vi "DPT File Setup.vi"(0 "Data File Directory":path=path "D:/Data", 1 "Test_Type:":string="HeatUP", 3 "Version In:":string="DGnn", 4 "Supply Voltage:":string(combo), 5 "error in (no error)":errorcluster, 7 "File Extension:":string="tmp", 12 "Scale Com Port":refnum<visa-resource-name>="COM1", 18 "Flow Computer Info Baro,BTUF,u,Z":string[][](array[string])) -> (11 "FileInit Cluster":T1={"Dryer Type"="NR", "TR Number"="", "Lab ID"="", "Output Stream Header"=[], "Stream Data Output"=[], "2015 Array"=[], "Dryer Test Data"=[], "Off Mode Array"=[], "Calibration Array"=[], "File Initialization Array"=[], "Load Run Number"="", "Model:"="DGnn", "Serial Number:"="DGnn", "Build:"="", "Test_Title Per TR:"="HeatUP", "Ambient Temp SetPoint:"="70", "Washer Water \nTemperature ( 60 ± 5°F ):"="60", "Frequency:"="60 HZ", "Dryness Setting:"="", "Heat Setting:"="", "Ambient RH:"="50", "Drying Cycle:"="", "Exhaust:"="NR", "Comments:"="", "Technician:"="", "Engineer:"="CraigT.", "Water Hardness (PPM)"="60", "Empty Dryer Cold Weight"="HeatUP", "Date:"="DGnn", "Version:"="DGnn", "Computer:"="1A", "Load Type"="", "Nominal Load  Weight"="", "Weights Out"={"Measured IMC"=7.0, "Actual RMC"=7.0, "RMC (Desired)"=100.0, "Bone Dry Wt(lbs)"=7.0, "Tolerance(%)"=5.0}, "Test Station:"="1A", "Heat Setting:"="", "Dryness Setting:"="", "Frequency:"="60 HZ", "Water Hardness (PPM)"="60", "Washer Water \nTemperature ( 60 ± 5°F )"="60", "Flow Computer Info Baro,BTUF,u,Z"=[], "Filename"="", "Analog Voltage Data"=[]} {"Weights Out"."Tolerance(%)" format="%0#_6g"; "Weights Out"."Bone Dry Wt(lbs)" format="%03_6g"; "Weights Out"."RMC (Desired)" format="%0#_6g"; "Weights Out"."Actual RMC" format="%03_6g"; "Weights Out"."Measured IMC" format="%0#_6g"}, 13 "Weights Out":T4={"Measured IMC"=7.0, "Actual RMC"=7.0, "RMC (Desired)"=100.0, "Bone Dry Wt(lbs)"=7.0, "Tolerance(%)"=5.0} {"Tolerance(%)" format="%0#_6g"; "Bone Dry Wt(lbs)" format="%03_6g"; "RMC (Desired)" format="%0#_6g"; "Actual RMC" format="%03_6g"; "Measured IMC" format="%0#_6g"}, 14 "FileName":path, 17 "Nominal Load  Weight":string(combo), 19 "error out":errorcluster)   [LabVIEW 2016, in "File Setup.lvlib"]
uses:
  File Setup.lvlib
  DPT Global Test Variables.vi
  Type Definition/DPT Output Dryer Information.ctl
  Custom Pallet Controls/Custom Pallet String.ctl
  Custom Pallet Controls/Custom Pallet Forward.ctl
panel:
  out "Description":string="File Name Setup"
  in  "Water Hardness (PPM)":T2
  in  "Model:":T2="DGnn"
  in  "Ambient Temp SetPoint:":T2="70"
  in  "Test_Title Per TR:":T2="HeatUP"
  in  "Engineer:":T2="CraigT."
  in  "Technician:":T2
  in  "Comments:":string
  in  "Lab ID:":T2="DGnn"
  in  "TR Number:":T2="T000000"
  in  "Load Run Number:":T2="001"
  in  "Exhaust:":string(combo)="NR"
  in  "Drying Cycle:":string(combo)
  in  "OK":T3
  in  "Serial Number:":T2="DGnn"
  in  "Ambient RH:":T2="50"
  in  "Build:":string(combo)
  in  "Heat Setting:":T2
  in  "Dryness Setting:":T2
  in  "Frequency:":T2="60 HZ"
  in  "Washer Water \nTemperature ( 60 ± 5°F ):":T2="60"
  in  "Dryer Type":string(combo)
  in  "Tab Control":enum32{"Location Data", "Output Data"}(tab)
  out "Unhandled Error":errorcluster
  out "Filename":string
  in  "Load Definition File":path=path "c:/Work/Loads.ini"
  out "Version:":string="DGnn"
  out "Computer:":string="1A"
  in  "Read Scale for IMC":bool
  out "Load Type":string(combo)
  out "Date:":string="DGnn"
  in  "Test Station:":string="1A"
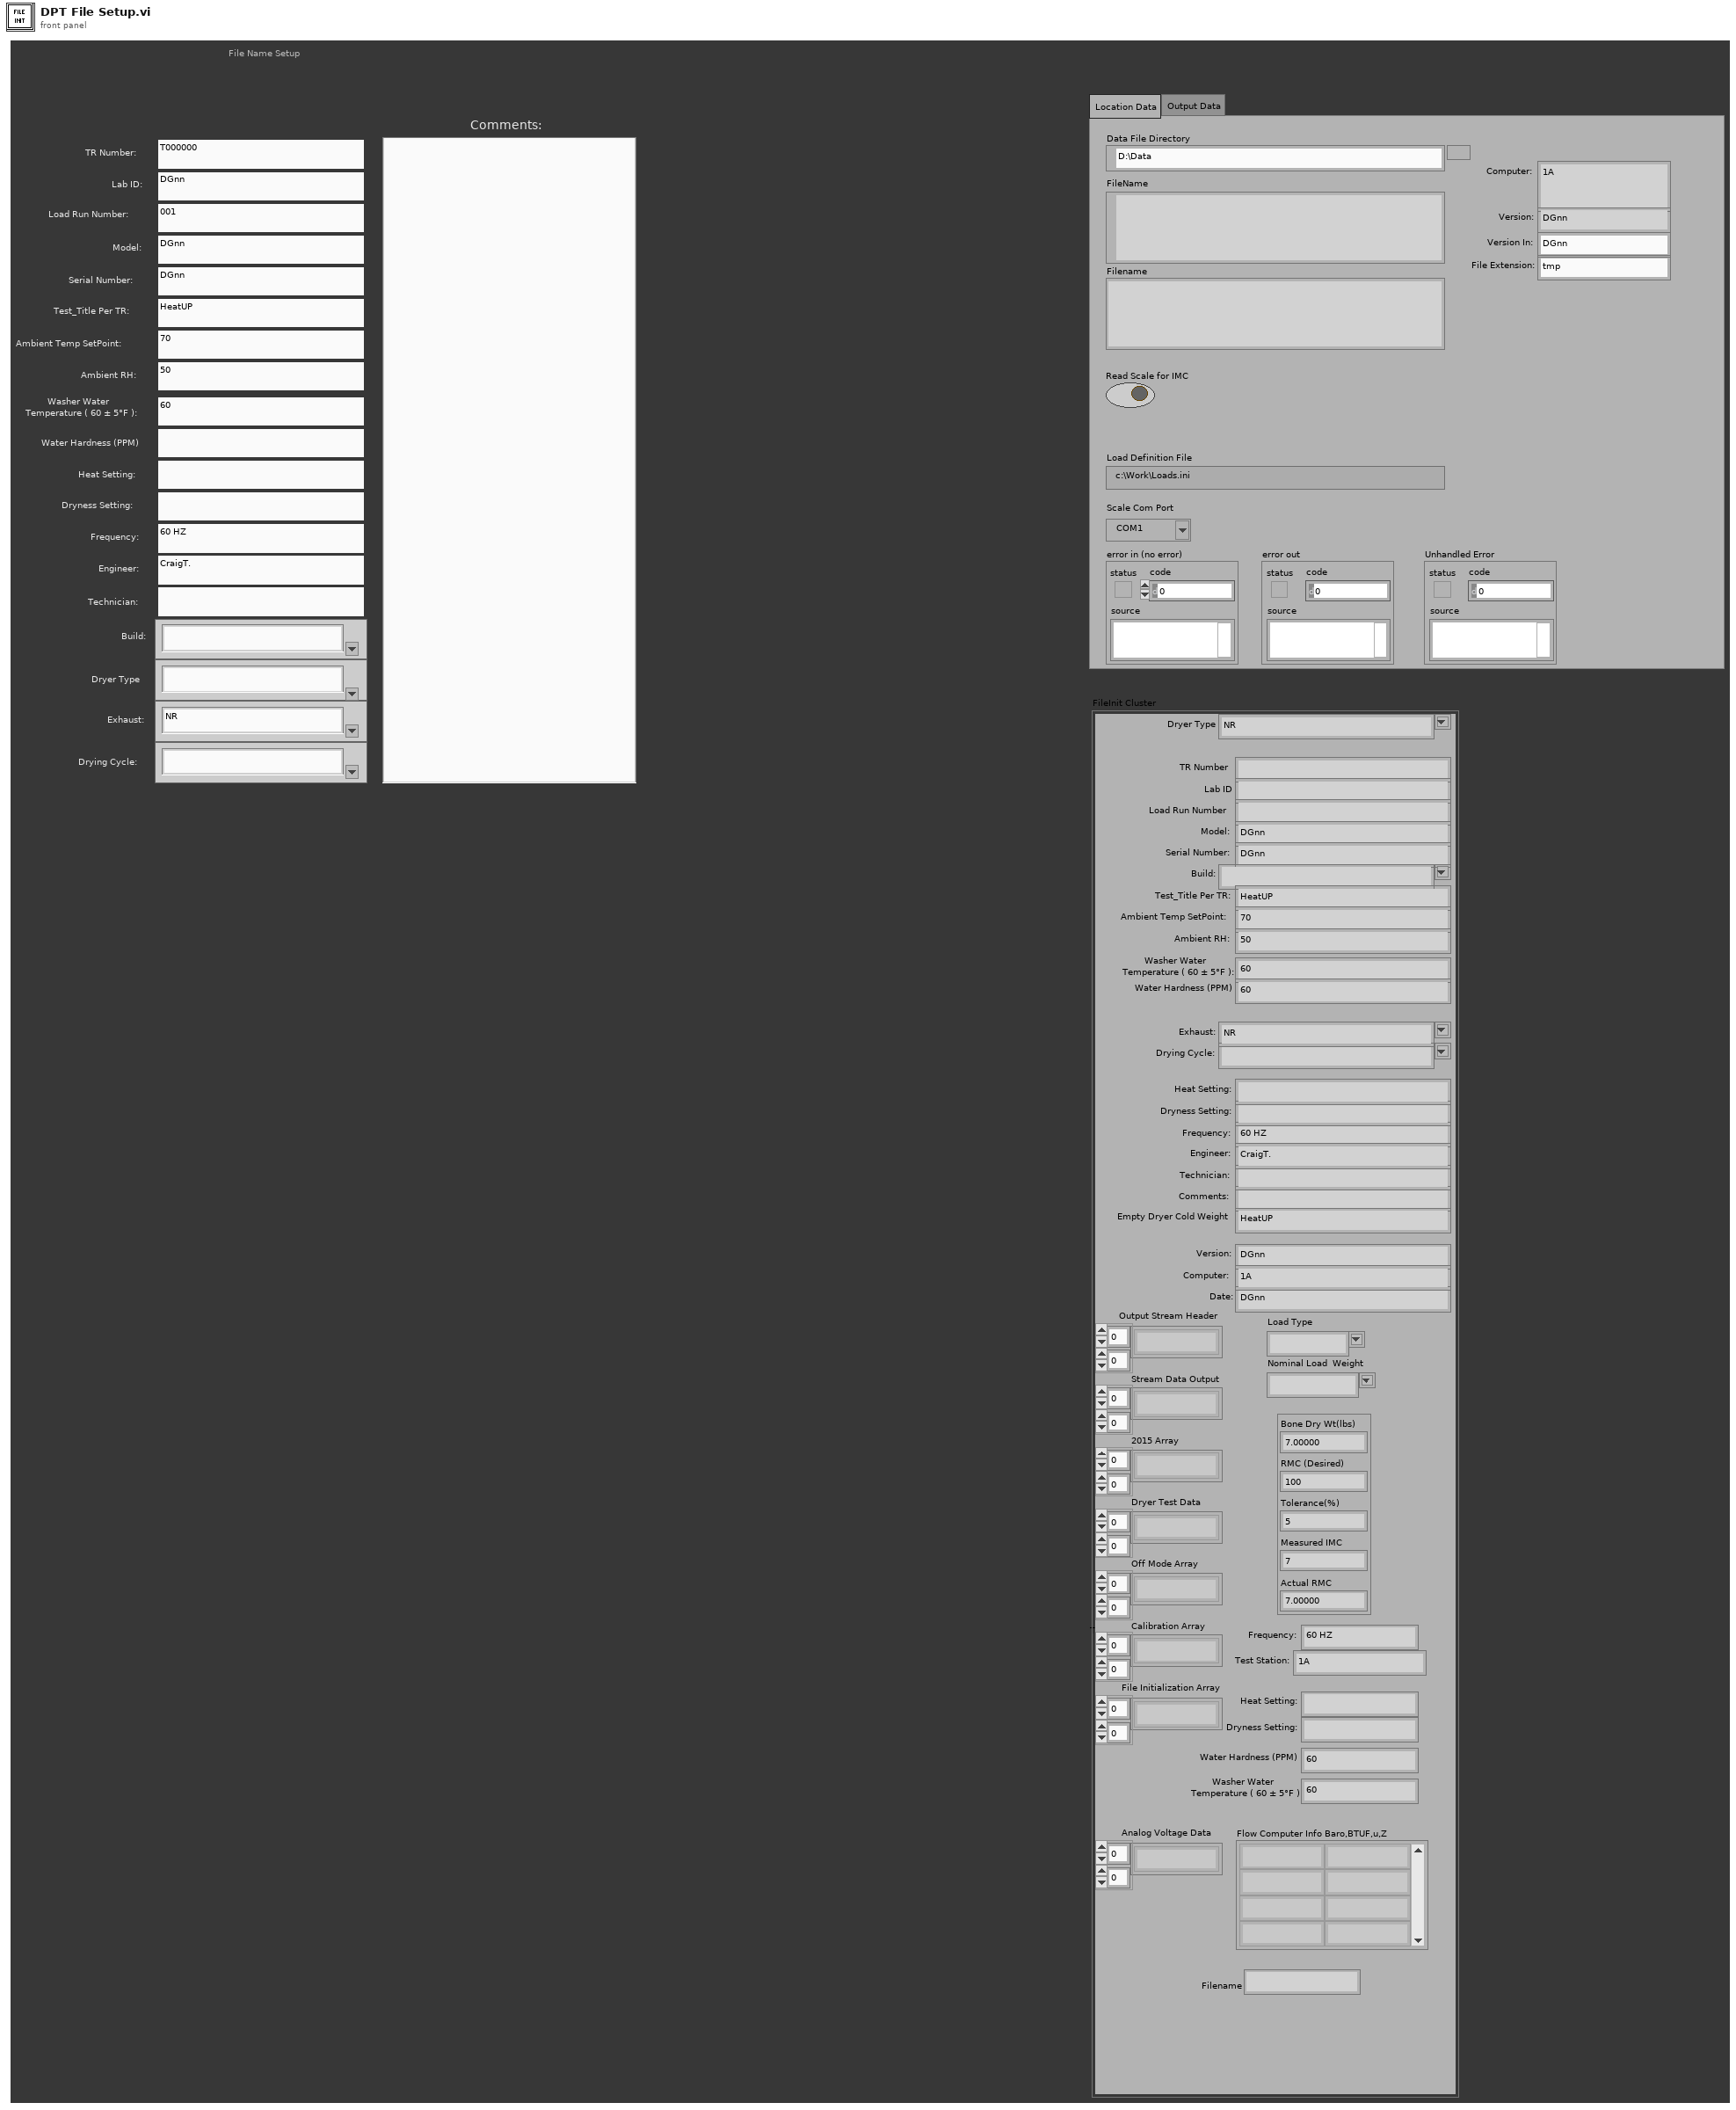
[diagram p1: front panel]
types:
  T1 = typedef "File Setup.lvlib/DPT Output Dryer Information.ctl" = cluster{"Dryer Type":string, "TR Number":string, "Lab ID":string, "Output Stream Header":string[][], "Stream Data Output":string[][], "2015 Array":string[][], "Dryer Test Data":string[][], "Off Mode Array":string[][], "Calibration Array":string[][], "File Initialization Array":string[][], "Load Run Number":string, "Model:":string, "Serial Number:":string, "Build:":string, "Test_Title Per TR:":string, "Ambient Temp SetPoint:":string, "Washer Water \nTemperature ( 60 ± 5°F ):":string, "Frequency:":string, "Dryness Setting:":string, "Heat Setting:":string, "Ambient RH:":string, "Drying Cycle:":string, "Exhaust:":string, "Comments:":string, "Technician:":string, "Engineer:":string, "Water Hardness (PPM)":string, "Empty Dryer Cold Weight":string, "Date:":string, "Version:":string, "Computer:":string, "Load Type":string, "Nominal Load  Weight":string, "Weights Out":cluster{"Measured IMC":dbl, "Actual RMC":dbl, "RMC (Desired)":dbl, "Bone Dry Wt(lbs)":dbl, "Tolerance(%)":dbl}, "Test Station:":string, "Heat Setting:":string, "Dryness Setting:":string, "Frequency:":string, "Water Hardness (PPM)":string, "Washer Water \nTemperature ( 60 ± 5°F )":string, "Flow Computer Info Baro,BTUF,u,Z":string[][], "Filename":string, "Analog Voltage Data":string[][]}
  T2 = typedef "Custom Pallet String.ctl" = string
  T3 = typedef "Custom Pallet Forward.ctl" = bool
  T4 = cluster{"Measured IMC":dbl, "Actual RMC":dbl, "RMC (Desired)":dbl, "Bone Dry Wt(lbs)":dbl, "Tolerance(%)":dbl}
  T5 = enum32{"invalid app kind", "Development System", "Run Time System", "Student Edition", "Embedded LabVIEW", "Evaluation", "Custom"}
  T6 = enum32{"Invalid", "Standard", "Closed", "Hidden", "Minimized", "Maximized"}
  T7 = cluster{"Core":cluster{"Current VI Reference":refnum<vi>, "Close Panel on Exit?":bool}, "Error Flag":bool, "Weights":cluster{"Measured IMC":dbl, "Actual RMC":dbl, "RMC (Desired)":dbl, "Bone Dry Wt(lbs)":dbl, "Tolerance(%)":dbl}, "Local?":bool, "Output Dryer Information":T1, "Test_Type:":string, "Supply Voltage:":string}
  T8 = cluster{"Current VI Reference":refnum<vi>, "Close Panel on Exit?":bool}
  T9 = typedef "File Setup.lvlib/DPT Global Type.ctl" = cluster{"Test Setup":cluster{"RH Resistor":dbl, "Temp Cal":dbl, "Temp Coeff":dbl, "Power On Threshold":dbl, "MA Filter Size":i32, "Weight Offset":dbl, "Temp Resistor":dbl, "Gas Enabled":bool, "Gas P. Resistor":dbl, "Scale Com":dbl, "W. Samps":i32, "Temp4mA Val":dbl, "Temp20mA Val":dbl, "RH4mA Val":dbl, "RH20mA Val":dbl, "GPres4mA Val":dbl, "Gpres20mA Val":dbl, "Smoothing":bool, "CDAQ":bool, "34970":bool, "34980":bool, "RH-IP":string, "RH-IP2":string, "RH-IP3":string, "CompVolume":dbl, "T45_Coeff.":dbl}, "Agilent Setup":cluster{"Scale Channel":string, "TC Channels":string, "VDC Discrete Channels":string, "RH Chan":string, "Temp Chan":string, "Tscale Channel":string, "RDB Channel":string, "Gas Temperature":string, "Gas Pressure":string, "Barometric Pressure":string, "Gas Feedback Chan":string}, "Directories":cluster{"Work File Directory":path, "Save File Directory":path, "Library Directory":path, "Data Backup Directory":path, "Data Backup Dir Fail":path, "Lab Directory":path}, "Test Information":cluster{"Model:":string, "Temperature:":string, "Engineer:":string, "Technician:":string, "Comments:":string, "Lab ID:":string, "TR Number:":string, "Test Number:":string, "Test Station:":string, "Empty Dryer Cold Weight:":dbl, "Serial Number:":string, "Build:":string, "Dryer Type":string, "Humidity":string, "Test Title per TR:":string}, "cDAQ Array Locations":cluster{"Scale Channel":string, "TC Channels":string, "VDC Discrete Channel":string, "RH Chan":string, "Temp Chan":string, "Tscale Channel":string, "RDB Channel":string, "Gas Temperature":string, "Gas Pressure":string, "Barometric Pressure":string, "Gas Feedback Chan":string}}
  T10 = cluster{"Model:":string, "Temperature:":string, "Engineer:":string, "Technician:":string, "Comments:":string, "Lab ID:":string, "TR Number:":string, "Test Number:":string, "Test Station:":string, "Empty Dryer Cold Weight:":dbl, "Serial Number:":string, "Build:":string, "Dryer Type":string, "Humidity":string, "Test Title per TR:":string}
  T11 = typedef "DPT IMC Data.ctl" = cluster{"Measured IMC (lbs)":dbl, "Actual Initial RMC (%)":dbl, "RMC (Desired %)":dbl, "Bone Dry Wt(lbs)":dbl, "Tolerance(%)":dbl, "Actual Final RMC (%)":dbl, "CEF (lbf/kWh)":dbl, "Minimum Weight (lbf)":dbl, "Average Weight (lbf)":dbl, "Maximum Weight (lbf)":dbl, "Measured IMC In Range?":bool, "Moisture Reduction Factor":dbl, "Field Use Factor":dbl, "Empty Dryer Cold Weigth":dbl, "Energy Standard":T12, "Weight Cloth (lbs)":dbl, "Relative Moisture Content (%)":dbl, "Relative Moisture Content - Avg (%)":dbl}
  T12 = typedef "DOE Dryer Standard.ctl" = enum16{"D2-Automatic Dryer", "D2-Timer Dryer", "D1-Automatic Dryer", "D1-Timer Dryer", "Other"}
  T13 = typedef "File Setup.lvlib/DPT Audit Data.ctl" = cluster{"Technician":string, "Date":string, "Model":string, "Serial":string, "Total Dry Time(m)":dbl, "Bone Dry Wt":dbl, "Initial Wt":dbl, "Final Wt":dbl, "Initial Ret":dbl, "Final Ret":dbl, "Elect Energy Used":dbl, "Gas Meter Temp":dbl, "Gas Meter Pres":dbl, "Gas Volume":dbl, "Barometer Temp":dbl, "Barometer Pres":dbl, "Gas Corr Fact":dbl, "Cor Gas Vol":dbl, "Gas Heat Val":dbl, "Gas Energy BTU":dbl, "Gas Energy kwh 4%":dbl, "Elect Energy kwh 4%":dbl, "Total  Energy 4%":dbl, "Gas Vol Init":dbl, "Gas Vol Fin":dbl, "Start Time(s)":dbl, "End Time(s)":dbl, "Elect Energy Start":dbl, "Elect Energy End":dbl, "Per Cycle Efficency":dbl, "Annual Consumption":dbl, "Load Cycles":string, "Ambinet Temp":string, "Ambinet RH":string, "Per Cycle Off Mode/Standby Power":dbl, "Total Energy (Gas + Elect)":dbl, "Combined Energy Factor":dbl, "Off Mode Power":dbl, "Exhaust":string, "Washer Water Temperature ( 60 ± 5°F )":string, "Supply Voltage":string, "Reference Temperature (F)":string, "Reference Pressure (psi)":string, "Standby Power":dbl}
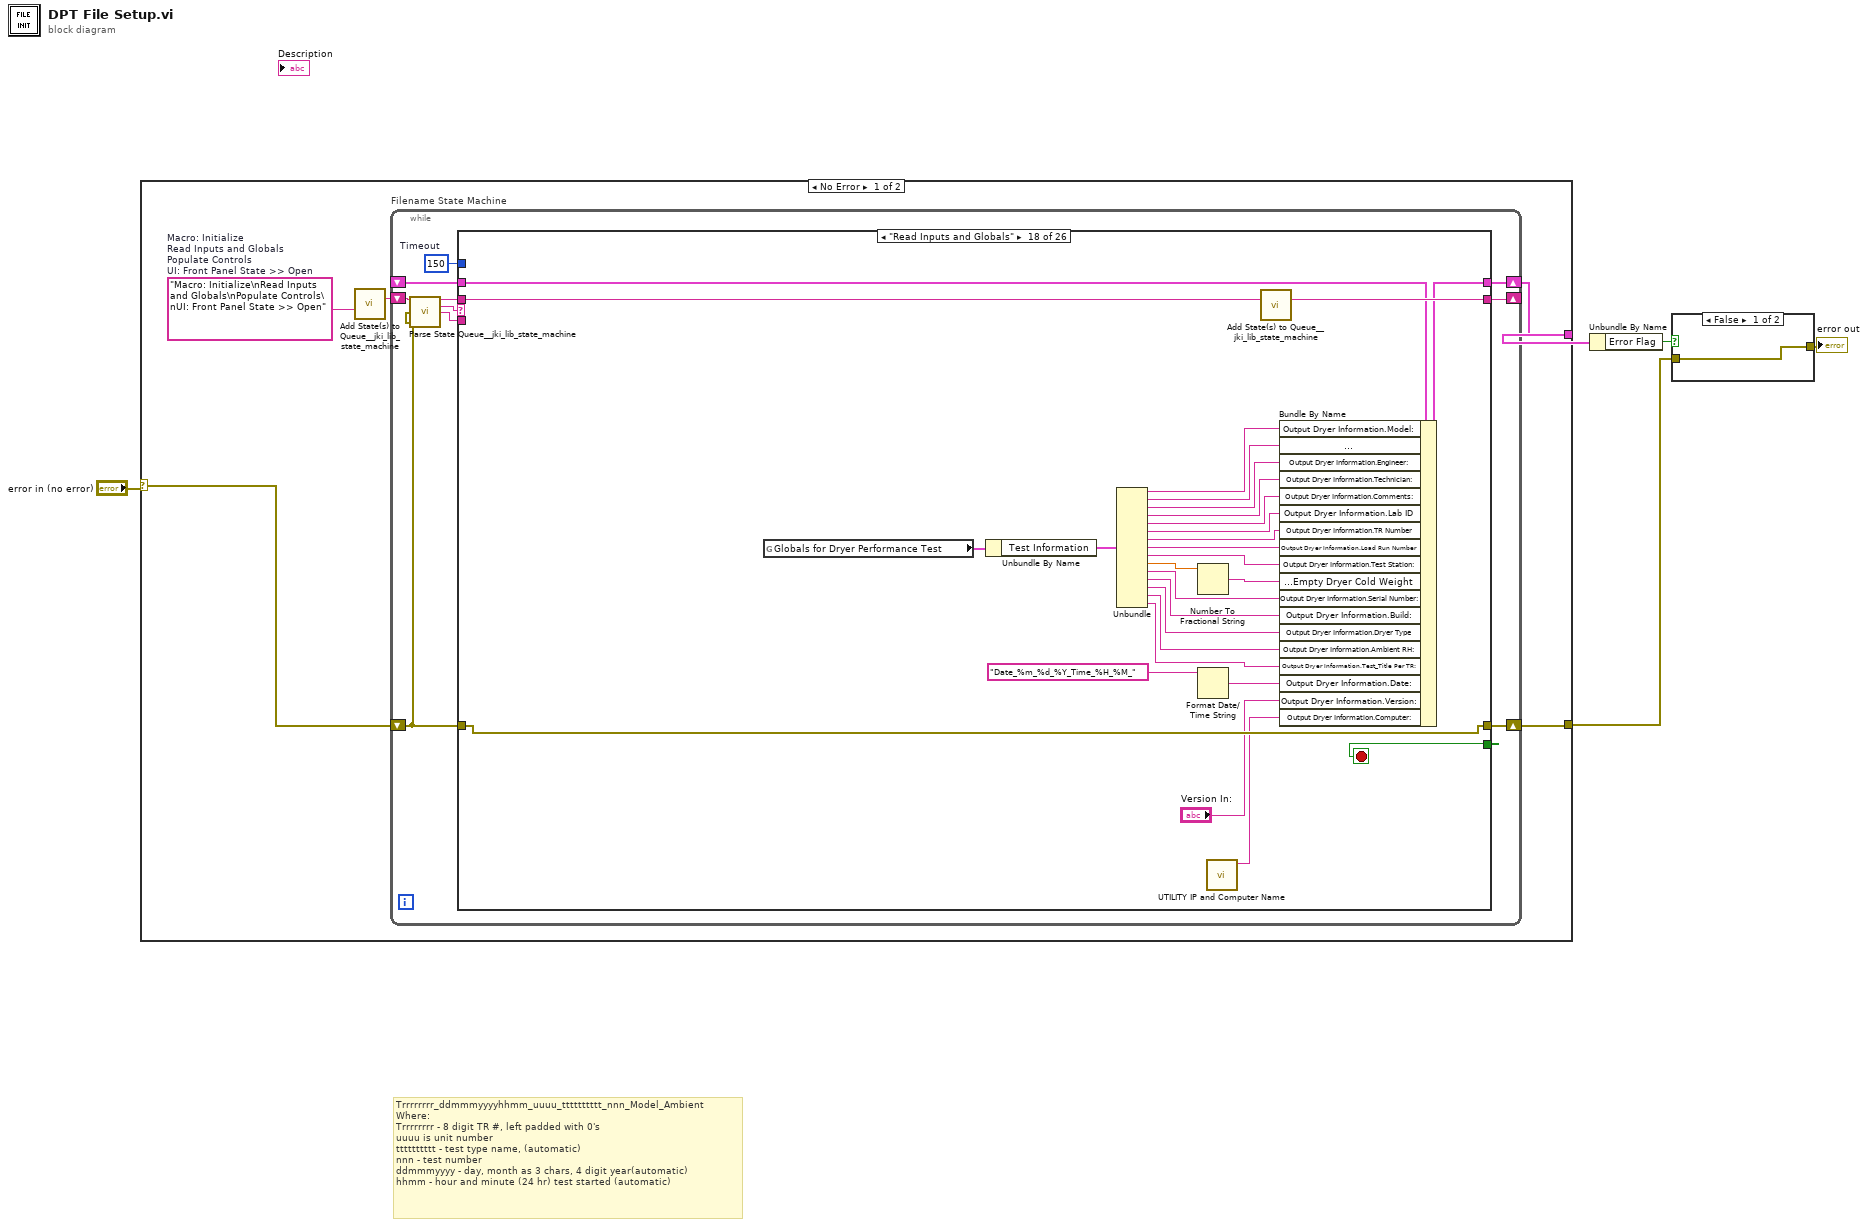
[diagram p0: block diagram]
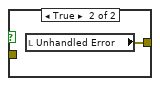
[diagram p2: hidden frame]
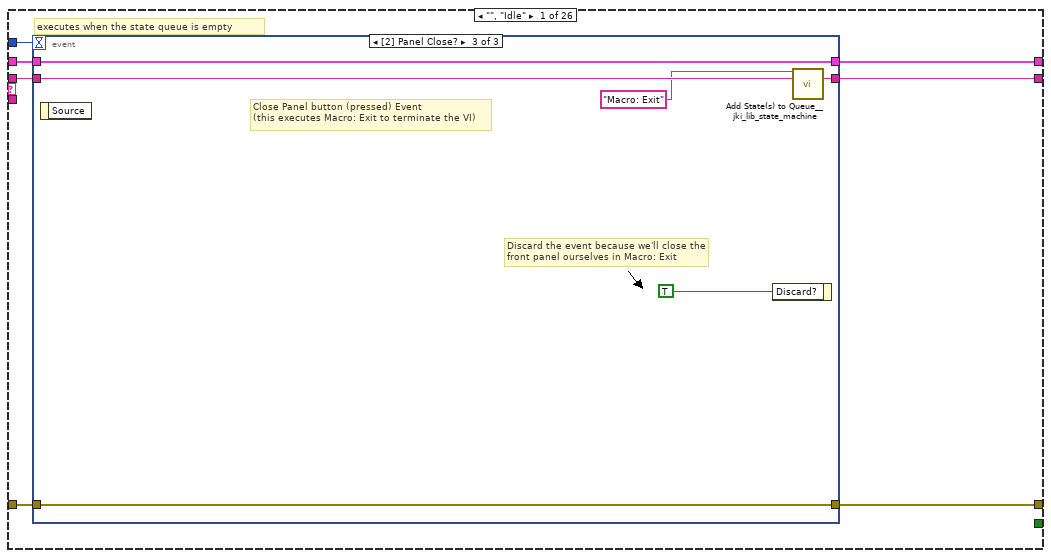
[diagram p3: hidden frame]
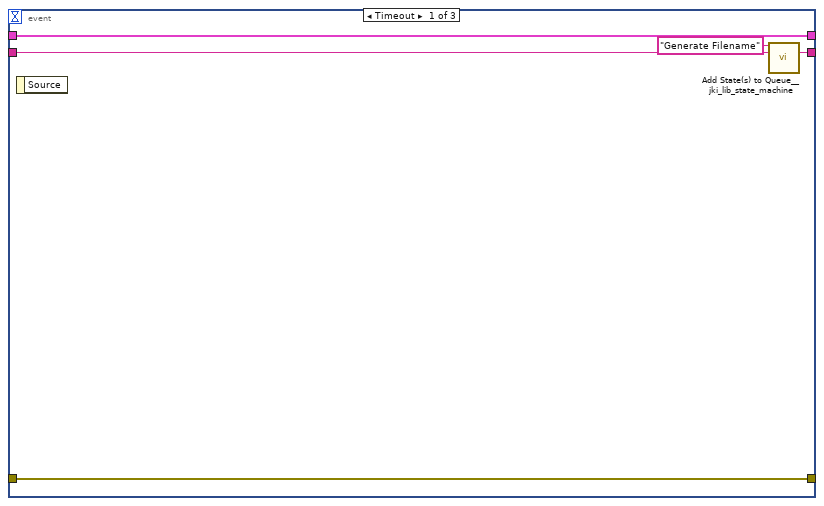
[diagram p4: hidden frame]
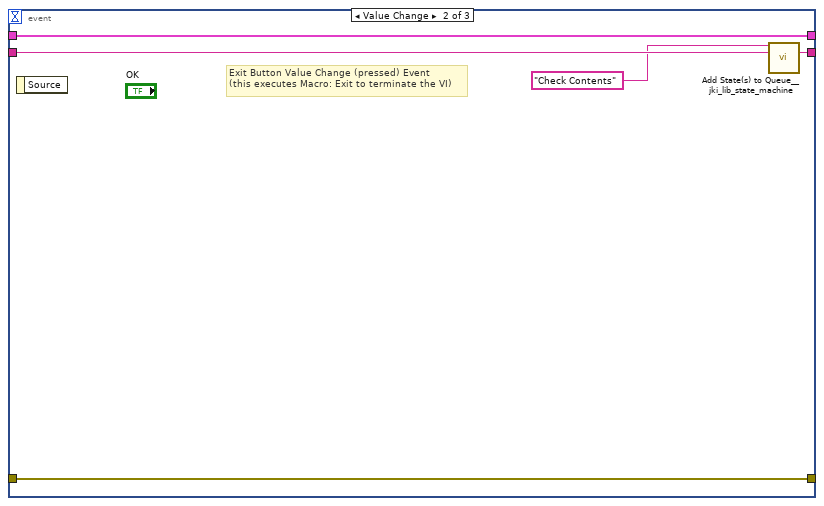
[diagram p5: hidden frame]
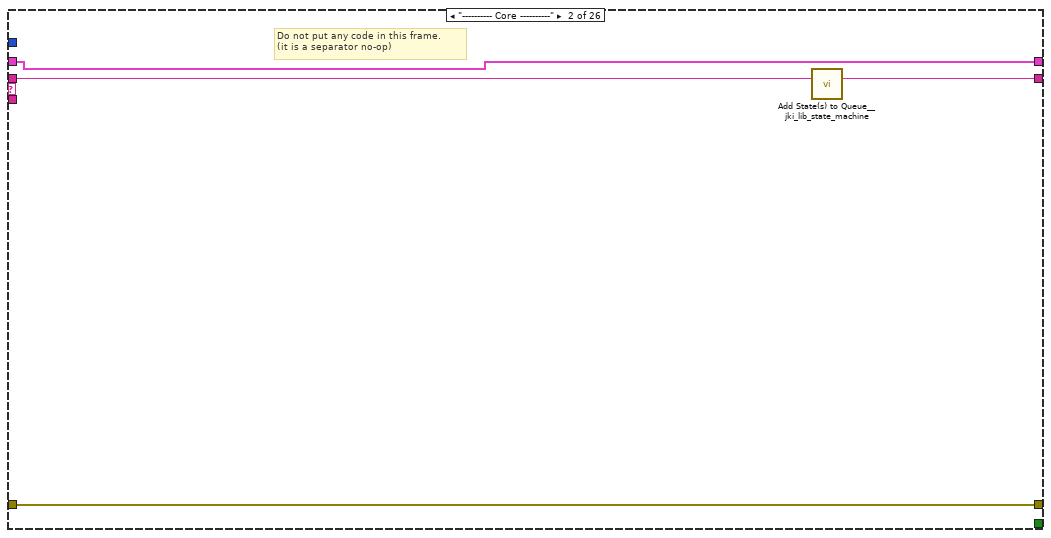
[diagram p6: hidden frame]
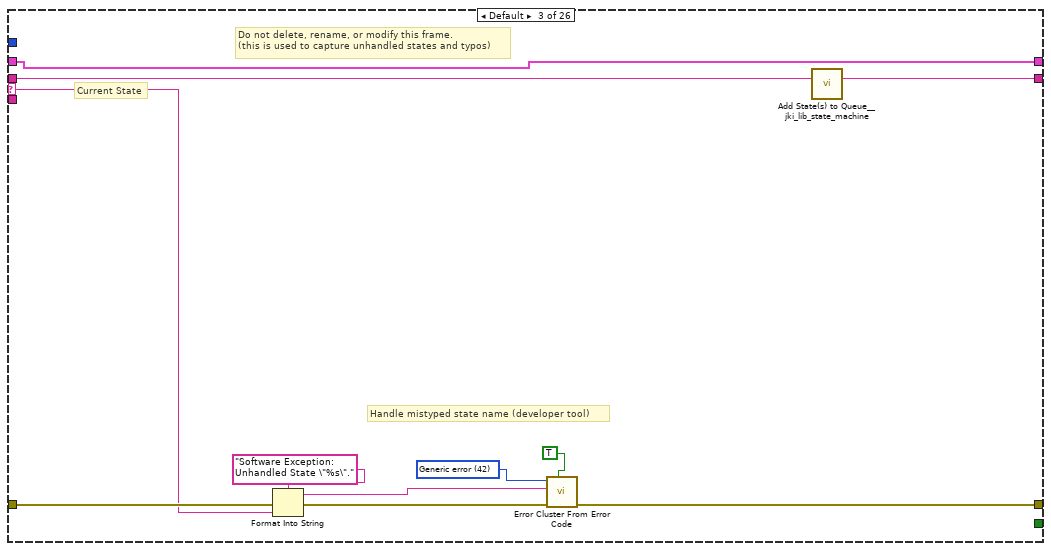
[diagram p7: hidden frame]
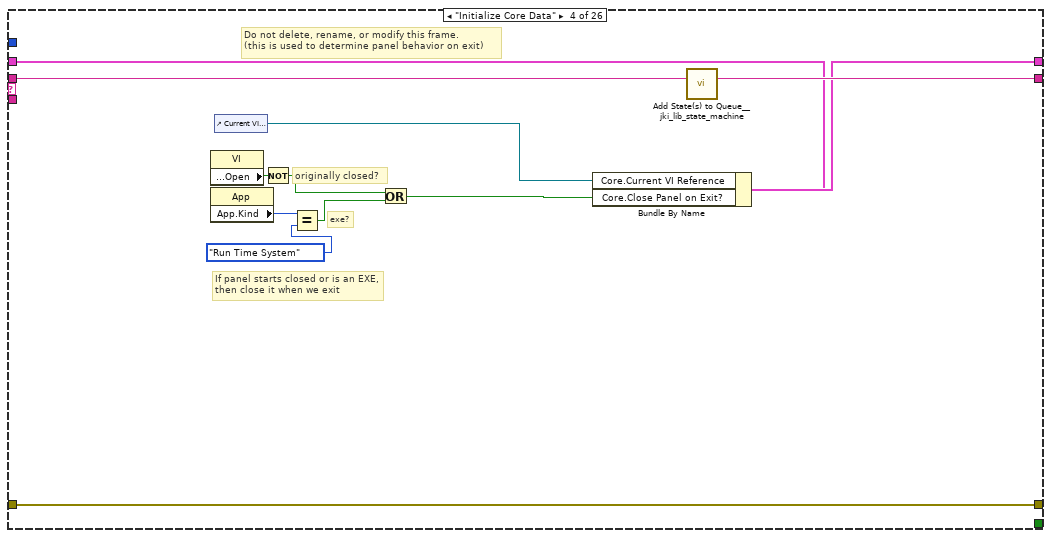
[diagram p8: hidden frame]
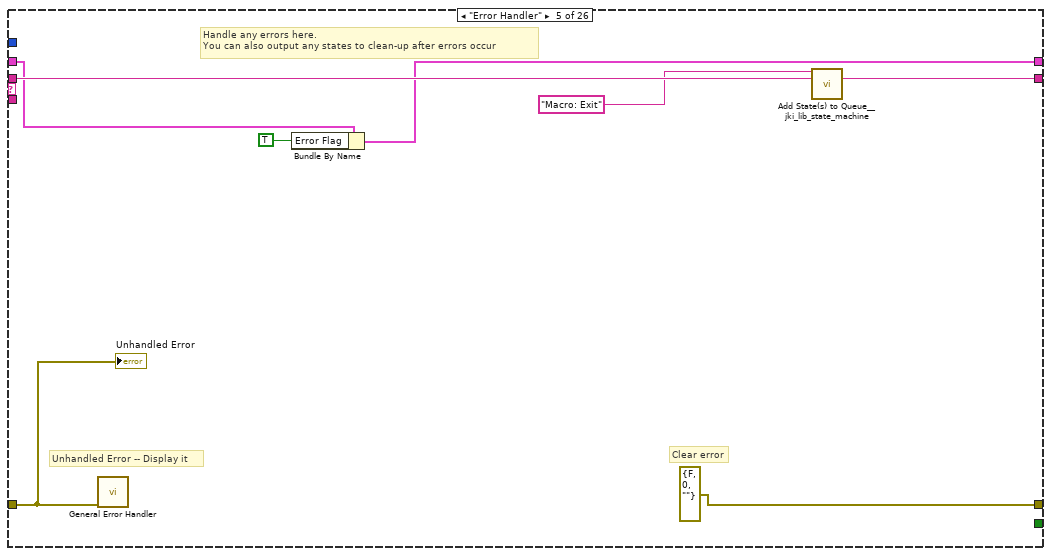
[diagram p9: hidden frame]
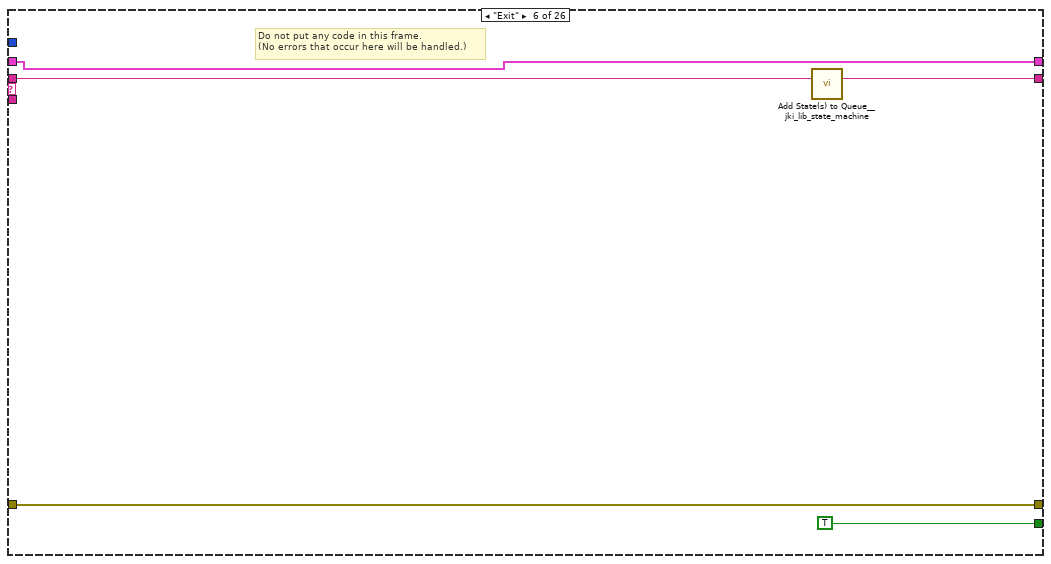
[diagram p10: hidden frame]
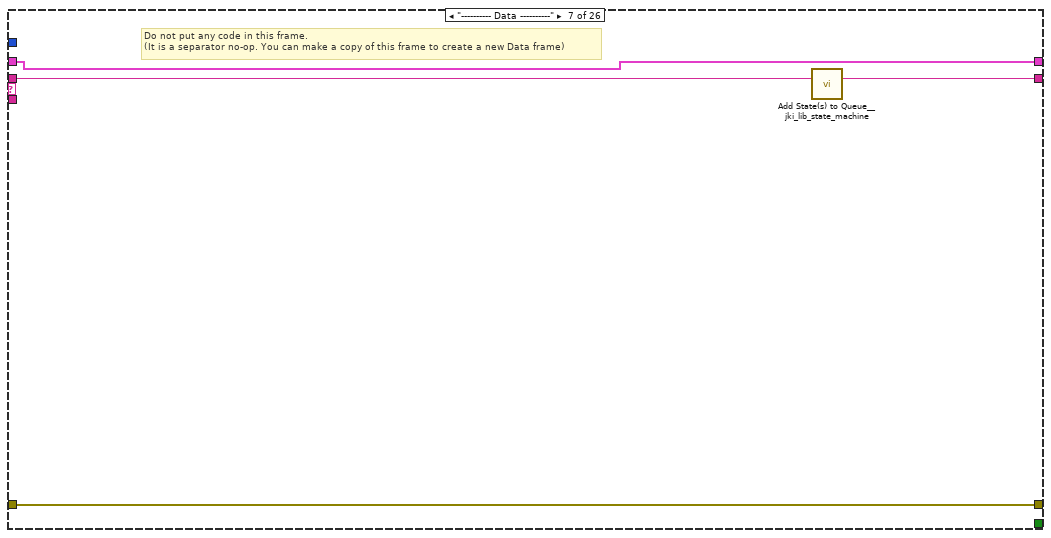
[diagram p11: hidden frame]
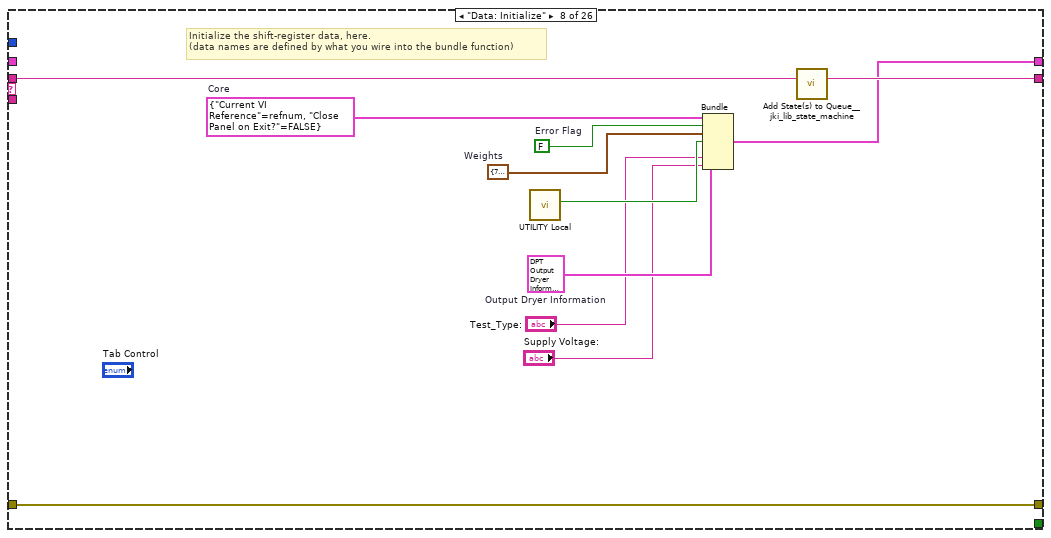
[diagram p12: hidden frame]
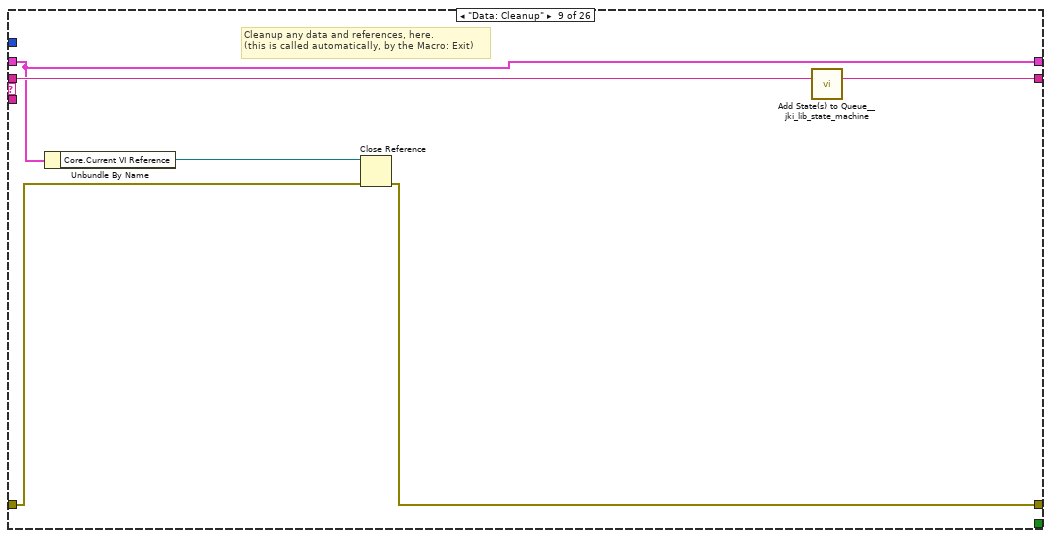
[diagram p13: hidden frame]
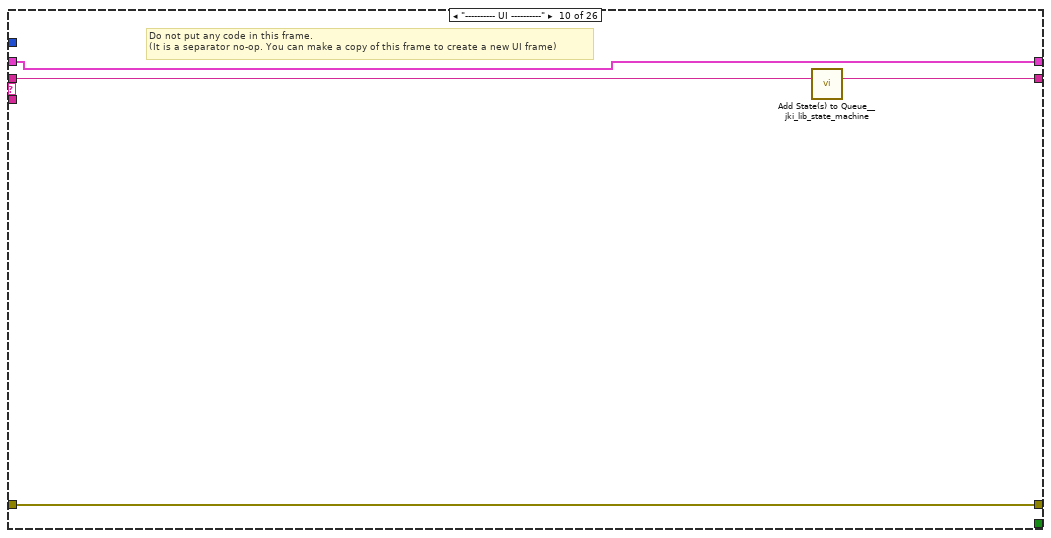
[diagram p14: hidden frame]
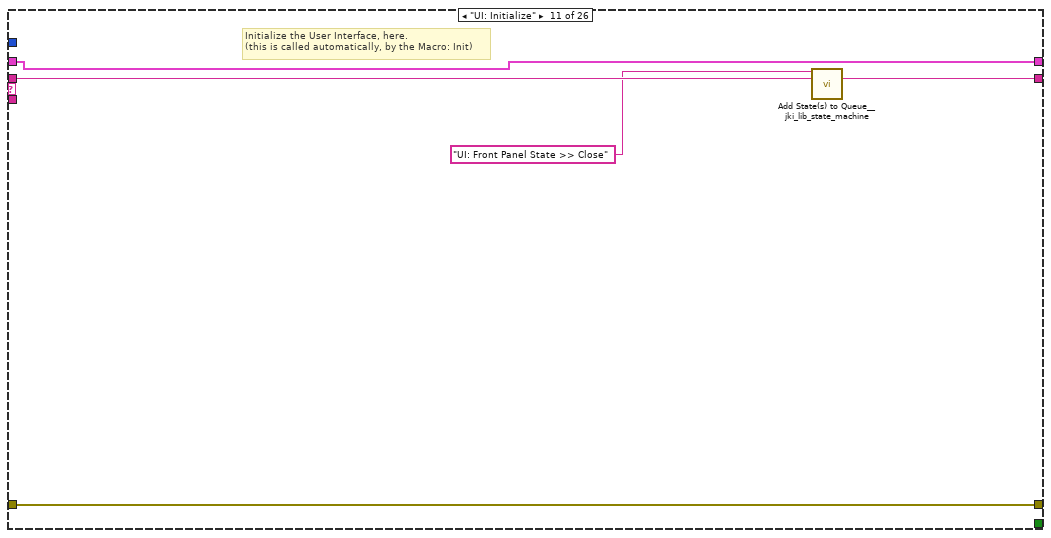
[diagram p15: hidden frame]
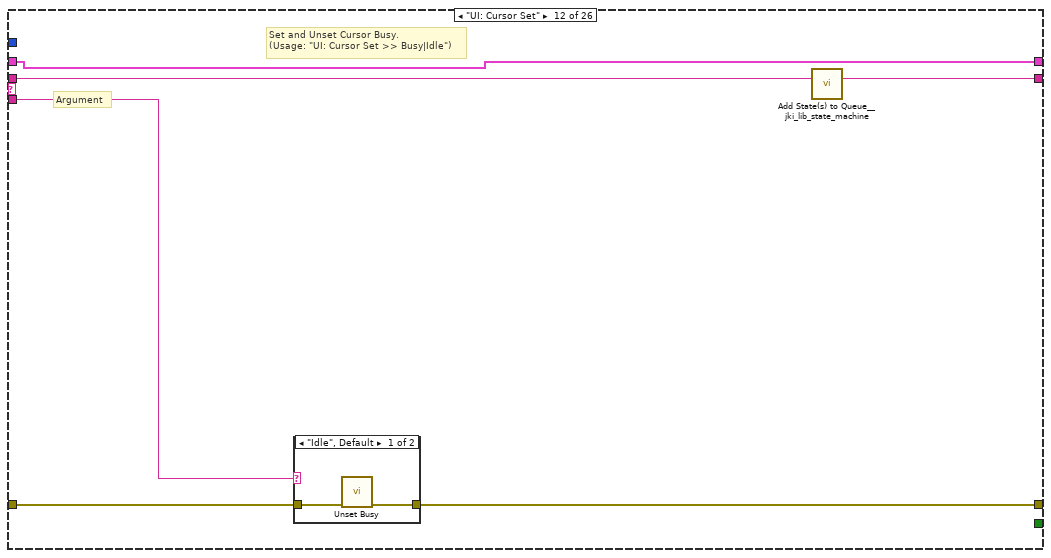
[diagram p16: hidden frame]
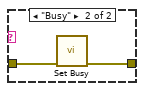
[diagram p17: hidden frame]
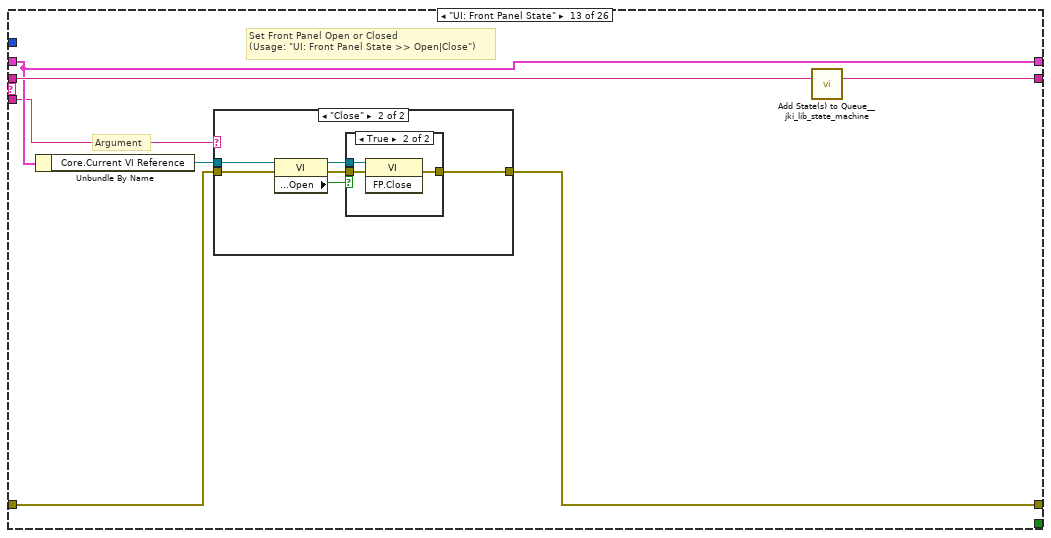
[diagram p18: hidden frame]
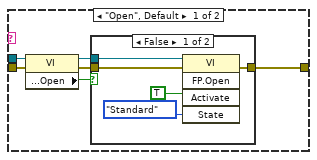
[diagram p19: hidden frame]
diagram:
  # "Trrrrrrrr_ddmmmyyyyhhmm_uuuu_tttttttttt_nnn_Model_Ambient\nWhere:\nTrrrrrrrr - 8 digit TR #, left padded with 0's\nuuuu is unit number\ntttttttttt - test type name, (automatic)\nnnn - test number\nddmmmyyyy - day, month as 3 chars, 4 digit year(automatic)\nhhmm - hour and minute (24 hr) test started (automatic)"
  n1 = case shown="No Error" "error in (no error)" {
    selector: "error in (no error)" -> [w7 w386]
    tunnel: [w8 _] -> w4
    tunnel: [w6 w386] -> w1
    frame No Error {
      w9 = "Macro: Initialize\nRead Inputs and Globals\nPopulate Controls\nUI: Front Panel State >> Open"  # Macro: Initialize Read Inputs and Globals Populate Controls UI: Front Panel State >> Open
      n2 = call <vilib>:"Add State(s) to Queue__jki_lib_state_machine.vi"("State(s) in (\"\")"=w9) -> ("States Out"=w10:string)  [unwired: 14 in]
      n3 = while "Filename State Machine" {
        shift-right: [w14] -> w8
        shift-left: _ -> [w13]
        shift-right: [w17] -> w6
        shift-left: w7 -> [w11]
        shift-right: [w16] -> _
        shift-left: w10 -> [w18]
        stop <- w15 stop-if-true
        w12 = 150  # Timeout
        n4 = call <vilib>:"Parse State Queue__jki_lib_state_machine.vi"("State Queue"=w18, "Error In (no error)"=w11) -> ("Remaining States"=w20:string, "Current State"=w21:string, "Arguments"=w19:string)  [unwired: 11 in]
        n5 = case shown="\"Read Inputs and Globals\"" w21 {
          selector: w21 -> [_ _ w49 _ _ _ _ _ _ _ _ _ _ _ _ _ _ _ _ _ _ _ _ _ _ _]
          tunnel: w20 -> [w28 w48 w53 w71 w79 w84 w88 w99 w105 w109 w114 w120 w131 w157 w164 w176 w180 w207 w226 w251 w266 w291 w301 w332 w365 w385]
          tunnel: w19 -> [_ _ _ _ _ _ _ _ _ _ _ w115 w125 _ _ _ _ _ _ _ _ _ _ _ _ _]
          tunnel: w13 -> [w26 w45 w51 w62 w74 w82 w85 _ w100 w106 w112 w118 w127 w154 w161 w173 w177 w200 w223 w232 w281 w287 w293 w305 w342 w378]
          tunnel: [w25 w46 w55 w68 errorcluster {"status"=FALSE, "code"=0, "source"=""} ("error out") w81 w86 w96 w101 w107 w111 w116 w128 w155 w162 w174 w178 w205 w224 w249 w282 w289 w299 w322 w358 w383] -> w17
          tunnel: w11 -> [w24 w46 w54 w68 w76 w81 w86 w96 w102 w107 w111 w117 w129 w155 w162 w174 w178 w205 w224 w249 w282 w289 w299 w323 w359 w383]
          tunnel: [w27 w47 w52 w70 w78 w83 w87 w98 w104 w108 w113 w119 w130 w156 w163 w175 w179 w206 w225 w250 w283 w290 w300 w331 w364 w384] -> w16
          tunnel: [_ _ _ _ _ TRUE _ _ _ _ _ _ _ _ _ _ _ _ _ _ _ _ _ _ _ _] -> w15
          tunnel: [w23 w45 w51 w69 w73 w82 w85 w97 w100 w106 w112 w118 w127 w154 w161 w173 w177 w199 w223 w231 w280 w286 w298 w304 w339 w378] -> w14
          tunnel: w12 -> [w22 _ _ _ _ _ _ _ _ _ _ _ _ _ _ _ _ _ _ _ _ _ _ _ _ _]
          frame "", "Idle" {
            # "executes when the state queue is empty"
            n6 = event shown="[2] Panel Close?" {
              selector: _ -> [_ _ _]
              dyn-events: _ -> [_ _ _]
              timeout: w22 -> [_ _ _]
              tunnel: w28 -> [w33 w38 w44]
              tunnel: [w32 w37 w43] -> w27
              tunnel: w26 -> [w30 w35 w41]
              tunnel: [w31 w36 w42] -> w25
              tunnel: w24 -> [w31 w36 w42]
              tunnel: [w30 w35 w41] -> w23
              event Timeout {
                n7 = event-data() -> ()  [unwired: 1 in, 1 out]
                n8 = call <vilib>:"Add State(s) to Queue__jki_lib_state_machine.vi"("State(s) in Front (\"\")"="Generate Filename" ("State(s) in Front (\"\")"), "State(s) in (\"\")"=w33) -> ("States Out"=w32:string)  [unwired: 13 in]
              }
              event Value Change {
                # "Exit Button Value Change (pressed) Event\n(this executes Macro: Exit to terminate the VI)"
                n9 = event-data() -> ()  [unwired: 1 in, 1 out]
                n10 = call <vilib>:"Add State(s) to Queue__jki_lib_state_machine.vi"("State(s) in Front (\"\")"="Check Contents", "State(s) in (\"\")"=w38) -> ("States Out"=w37:string)  [unwired: 13 in]
              }
              event Panel Close? {
                # "Discard the event because we'll close the front panel ourselves in Macro: Exit"
                # "Close Panel button (pressed) Event\n(this executes Macro: Exit to terminate the VI)"
                n11 = event-data() -> ()  [unwired: 1 in, 1 out]
                n12 = event-data("Discard?"=TRUE) -> ()  [unwired: 1 in, 1 out]
                n13 = call <vilib>:"Add State(s) to Queue__jki_lib_state_machine.vi"("State(s) in Front (\"\")"="Macro: Exit", "State(s) in (\"\")"=w44) -> ("States Out"=w43:string)  [unwired: 13 in]
              }
            }
          }
          frame "---------- Core ----------" {
            # "Do not put any code in this frame.\n(it is a separator no-op)"
            n14 = call <vilib>:"Add State(s) to Queue__jki_lib_state_machine.vi"("State(s) in (\"\")"=w48) -> ("States Out"=w47:string)  [unwired: 14 in]
          }
          frame Default {
            w58 = 42 items=["No error", "Argument error", "Memory is full", "Out of zone", "End of file", "File already open", "Generic file I/O error", "File not found", "File permission error", "Disk is full", "Duplicate path", "Too many files open", "System feature not enabled", "Resource file not found", "Cannot add resource", "Resource not found", "Image not found", "Image memory error", "Pen does not exist", "Config type invalid", "Config token not found", "Config parse error", "Config memory error", "Bad external code format", "Bad external code offset", "External code not present", "Null window", "Destroy window error", "Null menu", "Print aborted", "Bad print record", "Print driver error", "Windows error during printing", "Memory error during printing", "Print dialog error", "Generic print error", "Invalid device refnum", "Device not found", "Device parameter error", "Device unit error", "Cannot open device", "Device call aborted", "Generic error", "Cancelled by user", "Object ID too low", "Object ID too high", "Object not in heap", "Unknown heap", "Unknown object (invalid DefProc)", "Unknown object (DefProc not in table)", "Message out of range", "Invalid (null) method", "Unknown message", "Manager call not supported", "Bad address", "Network operation in progress", "Network operation timed out", "Connection is busy", "Network attribute not supported", "Network error", "Address in use", "System out of memory", "Connection aborted", "Connection refused", "Not connected", "Already connected", "Connection closed", "Initialization error (interapplication manager)", "Bad occurrence", "Wait on unbound occurrence handler", "Occurrence queue overflow", "Datalog type conflict", "Unused", "Unrecognized type (interapplication manager)", "Memory corrupt", "Failed to make temporary DLL", "Old CIN version", "Drag socket not found", "Failed to load drop-object", "Failed to register OLE object", "Failed to release OLE object", "Format specifier type mismatch", "Unknown format specifier", "Too few format specifiers", "Too many format specifiers", "Scan failed", "Newer CIN version", "Error converting to variant", "Runtime menu error", "Password tampered", "Variant attribute not found", "Incompatible variant data type", "Event data is not available", "Event Store is not present", "Occurrence is not found", "Event Queue is not created", "Event info is not available", "Refnum passed is NULL", "Error retrieving Class GUID", "Error retrieving CoClass GUID", "Error retrieving TypeLib GUID.", "Bad built application magic bytes.", "Specific driver is different from the specific driver associated with the Logical Name.", "There is no session opened to the class driver.", "Max Error", "MAX - Error with config objects", "MAX - Error loading configuration", "MAX - Group not supported"]
            # "Current State"
            # "Do not delete, rename, or modify this frame.\n(this is used to capture unhandled states and typos)"
            # "Handle mistyped state name (developer tool)"
            n15 = Format Into String(format string="Software Exception: Unhandled State \"%s\"." ("message"), error in=w54, w49) -> (resulting string=w57:string, error out=w56:errorcluster)  [unwired: 1 in]
            n16 = call <vilib>:"Error Cluster From Error Code.vi"("show call chain? (False)"=TRUE, "error in (no error)"=w56, "error message (\"\")"=w57, "error code (0)"=w58) -> ("error out"=w55:errorcluster)  [unwired: 5 in]
            n17 = call <vilib>:"Add State(s) to Queue__jki_lib_state_machine.vi"("State(s) in (\"\")"=w53) -> ("States Out"=w52:string)  [unwired: 14 in]
          }
          frame "Initialize Core Data" {
            # "Do not delete, rename, or modify this frame.\n(this is used to determine panel behavior on exit)"
            # "originally closed?"
            # "exe?"
            # "If panel starts closed or is an EXE, then close it when we exit"
            n18 = property class="VI"() -> ("Front Panel.Open"=w67:bool)  [unwired: 2 in, 2 out]
            n19 = property class="App"() -> ("App.Kind"=w66:T5)  [unwired: 2 in, 2 out]
            n20 = control-ref of="Current VI Reference"() -> (w60:refnum<vi>)
            n21 = Not(x=w67) -> (.not. x?=w64:bool)
            n22 = Equal?(x=w66, y=T5."Run Time System" ("Application:Kind")) -> (x = y?=w63:bool)
            n23 = Or(x=w64, y=w63) -> (x .or. y?=w61:bool)
            n24 = Bundle By Name(cluster=w62, "Core.Current VI Reference"=w60, "Core.Close Panel on Exit?"=w61) -> (w69:T7)
            n25 = call <vilib>:"Add State(s) to Queue__jki_lib_state_machine.vi"("State(s) in (\"\")"=w71) -> ("States Out"=w70:string)  [unwired: 14 in]
          }
          frame "Error Handler" {
            # "Unhandled Error -- Display it"
            # "Handle any errors here.\nYou can also output any states to clean-up after errors occur"
            # "Clear error"
            n26 = call <vilib>:"General Error Handler.vi"("error in (no error)"=w76) -> ()  [unwired: 10 in, 5 out]
            n27 = Bundle By Name(cluster=w74, "Error Flag"=TRUE) -> (w73:T7)
            n28 = call <vilib>:"Add State(s) to Queue__jki_lib_state_machine.vi"("State(s) in Front (\"\")"="Macro: Exit", "State(s) in (\"\")"=w79) -> ("States Out"=w78:string)  [unwired: 13 in]
            "Unhandled Error" <- w76
          }
          frame "Exit" {
            # "Do not put any code in this frame.\n(No errors that occur here will be handled.)"
            n29 = call <vilib>:"Add State(s) to Queue__jki_lib_state_machine.vi"("State(s) in (\"\")"=w84) -> ("States Out"=w83:string)  [unwired: 14 in]
          }
          frame "---------- Data ----------" {
            # "Do not put any code in this frame.\n(It is a separator no-op. You can make a copy of this frame to create a new Data frame)"
            n30 = call <vilib>:"Add State(s) to Queue__jki_lib_state_machine.vi"("State(s) in (\"\")"=w88) -> ("States Out"=w87:string)  [unwired: 14 in]
          }
          frame "Data: Initialize" {
            w91 = T1 {"Dryer Type"="NR", "TR Number"="", "Lab ID"="", "Output Stream Header"=[], "Stream Data Output"=[], "2015 Array"=[], "Dryer Test Data"=[], "Off Mode Array"=[], "Calibration Array"=[], "File Initialization Array"=[], "Load Run Number"="", "Model:"="", "Serial Number:"="", "Build:"="", "Test_Title Per TR:"="", "Ambient Temp SetPoint:"="", "Washer Water \nTemperature ( 60 ± 5°F ):"="", "Frequency:"="", "Dryness Setting:"="", "Heat Setting:"="", "Ambient RH:"="", "Drying Cycle:"="", "Exhaust:"="", "Comments:"="", "Technician:"="", "Engineer:"="", "Water Hardness (PPM)"="", "Empty Dryer Cold Weight"="", "Date:"="", "Version:"="", "Computer:"="", "Load Type"="", "Nominal Load  Weight"="", "Weights Out"={"Measured IMC"=0.0, "Actual RMC"=0.0, "RMC (Desired)"=0.0, "Bone Dry Wt(lbs)"=0.0, "Tolerance(%)"=0.0}, "Test Station:"="", "Heat Setting:"="", "Dryness Setting:"="", "Frequency:"="", "Water Hardness (PPM)"="", "Washer Water \nTemperature ( 60 ± 5°F )"="", "Flow Computer Info Baro,BTUF,u,Z"=[], "Filename"="", "Analog Voltage Data"=[]}  # Output Dryer Information
            w93 = T4 {"Measured IMC"=7.0, "Actual RMC"=7.0, "RMC (Desired)"=100.0, "Bone Dry Wt(lbs)"=7.0, "Tolerance(%)"=5.0}  # Weights
            w94 = T8 {"Current VI Reference"=refnum, "Close Panel on Exit?"=FALSE}  # Core
            w95 = FALSE  # Error Flag
            # "Initialize the shift-register data, here.\n(data names are defined by what you wire into the bundle function)"
            n31 = call "UTILITY Local.vi"() -> ("Local?"=w92:bool)  [unwired: 11 in]
            n32 = Bundle("Core"=w94, "Error Flag"=w95, "Weights"=w93, "Local?"=w92, "Output Dryer Information"=w91, "Test_Type:"="Test_Type:", "Supply Voltage:"="Supply Voltage:") -> (w97:T7)  [unwired: 1 in]
            n33 = call <vilib>:"Add State(s) to Queue__jki_lib_state_machine.vi"("State(s) in (\"\")"=w99) -> ("States Out"=w98:string)  [unwired: 14 in]
          }
          frame "Data: Cleanup" {
            # "Cleanup any data and references, here.\n(this is called automatically, by the Macro: Exit)"
            n34 = Unbundle By Name(w100) -> ("Core.Current VI Reference"=w103:refnum<vi>)
            n35 = Close Reference(reference=w103, error in (no error)=w102) -> (error out=w101:errorcluster)
            n36 = call <vilib>:"Add State(s) to Queue__jki_lib_state_machine.vi"("State(s) in (\"\")"=w105) -> ("States Out"=w104:string)  [unwired: 14 in]
          }
          frame "---------- UI ----------" {
            # "Do not put any code in this frame.\n(It is a separator no-op. You can make a copy of this frame to create a new UI frame)"
            n37 = call <vilib>:"Add State(s) to Queue__jki_lib_state_machine.vi"("State(s) in (\"\")"=w109) -> ("States Out"=w108:string)  [unwired: 14 in]
          }
          frame "UI: Initialize" {
            # "Initialize the User Interface, here.\n(this is called automatically, by the Macro: Init)"
            n38 = call <vilib>:"Add State(s) to Queue__jki_lib_state_machine.vi"("State(s) in Front (\"\")"="UI: Front Panel State >> Close", "State(s) in (\"\")"=w114) -> ("States Out"=w113:string)  [unwired: 13 in]
          }
          frame "UI: Cursor Set" {
            # "Argument"
            # "Set and Unset Cursor Busy.\n(Usage: \"UI: Cursor Set >> Busy|Idle\")"
            n39 = case shown="\"Idle\", Default" w115 {
              tunnel: w117 -> [w122 w124]
              tunnel: [w121 w123] -> w116
              frame "Idle", Default {
                n40 = call <vilib>:"Unset Busy.vi"("error in (no error)"=w122) -> ("error out"=w121:errorcluster)  [unwired: 10 in]
              }
              frame "Busy" {
                n41 = call <vilib>:"Set Busy.vi"("error in (no error)"=w124) -> ("error out"=w123:errorcluster)  [unwired: 9 in, 1 out]
              }
            }
            n42 = call <vilib>:"Add State(s) to Queue__jki_lib_state_machine.vi"("State(s) in (\"\")"=w120) -> ("States Out"=w119:string)  [unwired: 14 in]
          }
          frame "UI: Front Panel State" {
            # "Argument"
            # "Set Front Panel Open or Closed\n(Usage: \"UI: Front Panel State >> Open|Close\")"
            n43 = Unbundle By Name(w127) -> ("Core.Current VI Reference"=w126:refnum<vi>)
            n44 = case shown="\"Close\"" w125 {
              tunnel: w129 -> [w135 w148]
              tunnel: [w137 w149] -> w128
              tunnel: w126 -> [w136 w146]
              frame "Open", Default {
                n45 = property class="VI"(reference=w136, error in=w135) -> (reference out=w133:refnum<vi>, error out=w134:errorcluster, "Front Panel.Open"=w132:bool)
                n46 = case shown="False" w132 {
                  tunnel: [w140 w143] -> w137
                  tunnel: w134 -> [w139 w143]
                  tunnel: w133 -> [w138 _]
                  frame False {
                    n47 = invoke class="VI" method="FP.Open"(reference=w138, error in=w139, "Activate"=TRUE, "State"=T6."Standard") -> (error out=w140:errorcluster)  [unwired: 1 in, 4 out]
                  }
                  frame True {
                  }
                }
              }
              frame "Close" {
                n48 = property class="VI"(reference=w146, error in=w148) -> (reference out=w145:refnum<vi>, error out=w147:errorcluster, "Front Panel.Open"=w144:bool)
                n49 = case shown="True" w144 {
                  tunnel: [w150 w153] -> w149
                  tunnel: w147 -> [w150 w152]
                  tunnel: w145 -> [_ w151]
                  frame False {
                  }
                  frame True {
                    n50 = invoke class="VI" method="FP.Close"(reference=w151, error in=w152) -> (error out=w153:errorcluster)  [unwired: 1 in, 2 out]
                  }
                }
              }
            }
            n51 = call <vilib>:"Add State(s) to Queue__jki_lib_state_machine.vi"("State(s) in (\"\")"=w131) -> ("States Out"=w130:string)  [unwired: 14 in]
          }
          frame "---------- Macro ----------" {
            # "Do not put any code in this frame.\n(It is a separator no-op. You can make a copy of this frame to create a new Macro frame)"
            n52 = call <vilib>:"Add State(s) to Queue__jki_lib_state_machine.vi"("State(s) in (\"\")"=w157) -> ("States Out"=w156:string)  [unwired: 14 in]
          }
          frame "Macro: Initialize" {
            w158 = "" ("Dryer Type:")
            # "Initialization Macro\n(This is called once, when the VI starts)"
            n53 = property on="OK" class="Bool"("Key Focus"=FALSE) -> ()  [unwired: 2 in, 2 out]
            n54 = local write "Exhaust:"(w158) -> ()
            n55 = local write "Drying Cycle:"(w158) -> ()
            n56 = local write "Dryer Type"(w158) -> ()
            n57 = local write "Build:"(w158) -> ()
            n58 = call <vilib>:"Add State(s) to Queue__jki_lib_state_machine.vi"("State(s) in Front (\"\")"="Data: Initialize\nInitialize Core Data\nUI: Initialize", "State(s) in (\"\")"=w164) -> ("States Out"=w163:string)  [unwired: 13 in]
          }
          frame "Macro: Exit" {
            # "Exit Macro\n(This is called once, when the VI exits)"
            n59 = Unbundle By Name(w173) -> ("Core.Close Panel on Exit?"=w172:bool, "Local?"=w165:bool)
            n60 = Compound Arithmetic op=AND(w172, invert w165) -> (w166:bool)
            n61 = Select(t="UI: Front Panel State >> Close", s=w166, f="") -> (s? t:f=w169:string)
            n62 = call <vilib>:"Add State(s) to Queue__jki_lib_state_machine.vi"("State(s) in (\"\")"=w169, "State(s) at Back (\"\")"="Data: Cleanup\nExit") -> ("States Out"=w167:string)  [unwired: 13 in]
            n63 = call <vilib>:"Add State(s) to Queue__jki_lib_state_machine.vi"("State(s) in Front (\"\")"=w167, "State(s) in (\"\")"=w176) -> ("States Out"=w175:string)  [unwired: 13 in]
          }
          frame "---------- New Category ----------" {
            # "Template Separator\n(You can make a copy of, or modify, this frame)"
            n64 = call <vilib>:"Add State(s) to Queue__jki_lib_state_machine.vi"("State(s) in (\"\")"=w180) -> ("States Out"=w179:string)  [unwired: 14 in]
          }
          frame "Read Inputs and Globals" {
            n65 = global read "DPT Global Test Variables.vi" "Globals for Dryer Performance Test"() -> (w204:T9)
            n66 = Unbundle By Name(w204) -> ("Test Information"=w203:T10)
            n67 = Unbundle(w203) -> ("Model:"=w198:string, "Temperature:"=w197:string, "Engineer:"=w196:string, "Technician:"=w195:string, "Comments:"=w194:string, "Lab ID:"=w193:string, "TR Number:"=w192:string, "Test Number:"=w191:string, "Test Station:"=w184:string, "Empty Dryer Cold Weight:"=w202:dbl, "Serial Number:"=w189:string, "Build:"=w188:string, "Dryer Type"=w187:string, "Humidity"=w186:string, "Test Title per TR:"=w185:string)
            n68 = Number To Fractional String(number=w202) -> (F-format string=w190:string)  [unwired: 3 in]
            n69 = Format Date/Time String(time format string (%c)="Date_%m_%d_%Y_Time_%H_%M_") -> (date/time string=w183:string)  [unwired: 2 out]
            n70 = call "UTILITY IP and Computer Name.vi"() -> ("Computer Name"=w181:string)  [unwired: 10 in, 1 out]
            n71 = call <vilib>:"Add State(s) to Queue__jki_lib_state_machine.vi"("State(s) in (\"\")"=w207) -> ("States Out"=w206:string)  [unwired: 14 in]
            n72 = Bundle By Name(cluster=w200, "Output Dryer Information.Model:"=w198, "Output Dryer Information.Ambient Temp SetPoint:"=w197, "Output Dryer Information.Engineer:"=w196, "Output Dryer Information.Technician:"=w195, "Output Dryer Information.Comments:"=w194, "Output Dryer Information.Lab ID"=w193, "Output Dryer Information.TR Number"=w192, "Output Dryer Information.Load Run Number"=w191, "Output Dryer Information.Test Station:"=w184, "Output Dryer Information.Empty Dryer Cold Weight"=w190, "Output Dryer Information.Serial Number:"=w189, "Output Dryer Information.Build:"=w188, "Output Dryer Information.Dryer Type"=w187, "Output Dryer Information.Ambient RH:"=w186, "Output Dryer Information.Test_Title Per TR:"=w185, "Output Dryer Information.Date:"=w183, "Output Dryer Information.Version:"="Version In:", "Output Dryer Information.Computer:"=w181) -> (w199:T7)
          }
          frame "Populate Controls" {
            n73 = Unbundle By Name(w223) -> ("Output Dryer Information.Model:"=w219:string, "Output Dryer Information.Ambient Temp SetPoint:"=w218:string, "Output Dryer Information.Engineer:"=w217:string, "Output Dryer Information.Technician:"=w216:string, "Output Dryer Information.Comments:"=w215:string, "Output Dryer Information.Lab ID"=w214:string, "Output Dryer Information.TR Number"=w213:string, "Output Dryer Information.Load Run Number"=w212:string, "Output Dryer Information.Test Station:"=w211:string, "Output Dryer Information.Serial Number:"=w210:string, "Output Dryer Information.Ambient RH:"=w209:string, "Output Dryer Information.Test_Title Per TR:"=w208:string, "Output Dryer Information.Date:"=→"Date:":string, "Output Dryer Information.Version:"=→"Version:":string, "Output Dryer Information.Computer:"=→"Computer:":string)  [unwired: 1 out]
            n74 = local write "Model:"(w219) -> ()
            n75 = local write "Ambient Temp SetPoint:"(w218) -> ()
            n76 = local write "Engineer:"(w217) -> ()
            n77 = local write "Technician:"(w216) -> ()
            n78 = local write "Comments:"(w215) -> ()
            n79 = local write "Lab ID:"(w214) -> ()
            n80 = local write "TR Number:"(w213) -> ()
            n81 = local write "Load Run Number:"(w212) -> ()
            n82 = local write "Test Station:"(w211) -> ()
            n83 = local write "Serial Number:"(w210) -> ()
            n84 = local write "Ambient RH:"(w209) -> ()
            n85 = local write "Test_Title Per TR:"(w208) -> ()
            n86 = call <vilib>:"Add State(s) to Queue__jki_lib_state_machine.vi"("State(s) in (\"\")"=w226) -> ("States Out"=w225:string)  [unwired: 14 in]
          }
          frame "Check Contents" {
            n87 = Equal?(x="Drying Cycle:", y="Timed Dry" ("Drying Cycle:")) -> (x = y?=w238:bool)
            n88 = case shown="True" w238 {
              frame False {
              }
              frame True {
                n89 = local write "Dryness Setting:"("NA" ("Dryness Setting:")) -> ()
              }
            }
            n90 = Unbundle By Name(w232) -> ("Local?"=w240:bool, "Supply Voltage:"=w233:string)
            n91 = String Length(string="Water Hardness (PPM)") -> (length=w235:i32)
            n92 = Greater Than 0?(x=w235) -> (x > 0?=w234:bool)
            n93 = String Length(string="Exhaust:") -> (length=w248:i32)
            n94 = String Length(string="Drying Cycle:") -> (length=w247:i32)
            n95 = String Length(string=w233) -> (length=w246:i32)
            n96 = String Length(string="Dryer Type") -> (length=w237:i32)
            n97 = Greater Than 0?(x=w248) -> (x > 0?=w243:bool)
            n98 = Greater Than 0?(x=w247) -> (x > 0?=w244:bool)
            n99 = Greater Than 0?(x=w246) -> (x > 0?=w245:bool)
            n100 = Greater Than 0?(x=w237) -> (x > 0?=w236:bool)
            n101 = Compound Arithmetic op=AND(w243, w244, w245, w236, w234) -> (w242:bool)
            n102 = case shown="True" w242 {
              tunnel: ["" w263] -> w241
              tunnel: w240 -> [_ w262]
              tunnel: w232 -> [w253 w261]
              tunnel: [w253 w260] -> w231
              tunnel: "Drying Cycle:" -> [_ w259]
              tunnel: "Exhaust:" -> [_ w258]
              tunnel: "Dryer Type" -> [_ w257]
              tunnel: "Water Hardness (PPM)" -> [_ w256]
              frame False {
                n103 = One Button Dialog(message="All Test Data Must be Filled In") -> ()  [unwired: 1 in, 1 out]
              }
              frame True {
                n104 = case shown="True" w262 {
                  tunnel: ["UI: Front Panel State >> Close\nGet New Info\nGet Load Definition\nGet Weights\nGenerate Filename\nGenerate Header Data\nWrite Globals\nMacro: Exit" "Get New Info\nGet Load Definition\nGet Weights\nGenerate Filename\nGenerate Header Data\nWrite Globals\nMacro: Exit"] -> w263
                  frame False {
                  }
                  frame True {
                  }
                }
                n105 = Bundle By Name(cluster=w261, "Output Dryer Information.Exhaust:"=w258, "Output Dryer Information.Drying Cycle:"=w259, "Output Dryer Information.Dryer Type"=w257, "Output Dryer Information.Water Hardness (PPM)"=w256) -> (w260:T7)
              }
            }
            n106 = call <vilib>:"Add State(s) to Queue__jki_lib_state_machine.vi"("State(s) in Front (\"\")"=w241, "State(s) in (\"\")"=w251) -> ("States Out"=w250:string)  [unwired: 13 in]
          }
          frame "Get New Info" {
            n107 = Bundle By Name(cluster=w281, "Output Dryer Information.Model:"="Model:", "Output Dryer Information.Ambient Temp SetPoint:"="Ambient Temp SetPoint:", "Output Dryer Information.Engineer:"="Engineer:", "Output Dryer Information.Technician:"="Technician:", "Output Dryer Information.Comments:"="Comments:", "Output Dryer Information.Lab ID"="Lab ID:", "Output Dryer Information.TR Number"="TR Number:", "Output Dryer Information.Load Run Number"="Load Run Number:", "Output Dryer Information.Test Station:"="Test Station:", "Output Dryer Information.Serial Number:"="Serial Number:", "Output Dryer Information.Build:"="Build:", "Output Dryer Information.Ambient RH:"="Ambient RH:", "Output Dryer Information.Test_Title Per TR:"="Test_Title Per TR:") -> (w280:T7)
            n108 = call <vilib>:"Add State(s) to Queue__jki_lib_state_machine.vi"("State(s) in (\"\")"=w266) -> ("States Out"=w283:string)  [unwired: 14 in]
          }
          frame "Get Load Definition" {
            # "Get the nominal weight from user"
            n109 = call "DPT Panel Get Load Info.vi"("file path (dialog if empty)"="Load Definition File") -> ("Load Type Out"=w285:string, "Nominal Load  Weight Out"=w284:string)  [unwired: 12 in, 1 out]
            "Load Type" <- w285
            "Nominal Load  Weight" <- w284
            n110 = Bundle By Name(cluster=w287, "Output Dryer Information.Load Type"=w285, "Output Dryer Information.Nominal Load  Weight"=w284) -> (w286:T7)
            n111 = call <vilib>:"Add State(s) to Queue__jki_lib_state_machine.vi"("State(s) in (\"\")"=w291) -> ("States Out"=w290:string)  [unwired: 14 in]
          }
          frame "Get Weights" {
            # "Get the actual IMC from either user input or scale"
            n112 = Unbundle By Name(w293) -> ("Output Dryer Information.Nominal Load  Weight"=w292:string)
            n113 = Fract/Exp String To Number(string=w292) -> (number=w296:dbl)  [unwired: 3 in, 1 out]
            n114 = call "DPT Panel RMC Calculator.vi"("Scale Com Port"="Scale Com Port", "Bone Dry Weight (lbs)"=w296, "Read Scale Weight"="Read Scale for IMC") -> ("DPT IMC Data Out"=w297:T11)  [unwired: 11 in, 1 out]
            "Weights Out" <- w297
            n115 = Bundle By Name(cluster=w293, "Output Dryer Information.Weights Out"=w297) -> (w298:T7)
            n116 = call <vilib>:"Add State(s) to Queue__jki_lib_state_machine.vi"("State(s) in (\"\")"=w301) -> ("States Out"=w300:string)  [unwired: 14 in]
          }
          frame "Generate Filename" {
            # "Generate the filename"
            n117 = Unbundle By Name(w305) -> ("Output Dryer Information.TR Number"=w315:string, "Output Dryer Information.Lab ID"=w314:string, "Output Dryer Information.Nominal Load  Weight"=w313:string, "Output Dryer Information.Load Type"=w312:string, "Output Dryer Information.Exhaust:"=w311:string, "Output Dryer Information.Weights Out.RMC (Desired)"=w310:dbl, "Output Dryer Information.Test Station:"=w302:string, "Output Dryer Information.Technician:"=w309:string, "Output Dryer Information.Load Run Number"=w308:string, "Output Dryer Information.Ambient Temp SetPoint:"=w307:string, "Output Dryer Information.Date:"=w306:string)
            n118 = Number To Fractional String(number=w310, width (-)=i16 2, precision (6)=i16 0) -> (F-format string=w329:string)  [unwired: 1 in]
            n119 = Format Into String(format string="TR_%s_Lab_ID_%s_Cloth_Weight_%slbs_%s_Exhaust_%s_IMC_%s_Test_Station_%s_%s_Run %s_AmbT_%s_%sDPT.%s", w315, w314, w313, w312, w311, w329, w302, w309, w308, w307, w306, "File Extension:") -> (resulting string=w303:string)  [unwired: 2 in, 1 out]
            "Filename" <- w303
            n120 = Path To String(path="Data File Directory") -> (string=w318:string)
            n121 = Build Path(base path="Data File Directory", name or relative path=w303) -> (appended path=w325:path)
            "FileName" <- w325
            n122 = Concatenate Strings("Error for Filename: " ("source"), w303, " Directory: " ("source"), w318) -> (w317:string)
            n123 = Equal?(x=w325, y=path "") -> (x = y?=w324:bool)
            n124 = case shown="False" w324 {
              tunnel: w323 -> [w333 _]
              tunnel: [w333 w335] -> w322
              tunnel: w317 -> [_ w334]
              frame False {
              }
              frame True {
                n125 = Bundle By Name(cluster=errorcluster {"status"=TRUE, "code"=-8074, "source"=""} ("error IO"), "source"=w334) -> (w335:errorcluster)
              }
            }
            n126 = call <vilib>:"Add State(s) to Queue__jki_lib_state_machine.vi"("State(s) in (\"\")"=w332) -> ("States Out"=w331:string)  [unwired: 14 in]
            n127 = Bundle By Name(cluster=w305, "Output Dryer Information.Filename"=w303) -> (w304:T7)
          }
          frame "Generate Header Data" {
            n128 = Unbundle By Name(w342) -> ("Output Dryer Information"=w356:T1, "Test_Type:"=w351:string, "Supply Voltage:"=w344:string)
            n129 = Unbundle By Name(w342) -> ("Output Dryer Information.Technician:"=w350:string, "Output Dryer Information.Date:"=w349:string, "Output Dryer Information.Model:"=w348:string, "Output Dryer Information.Serial Number:"=w347:string, "Output Dryer Information.Load Run Number"=w346:string, "Output Dryer Information.Exhaust:"=w345:string, "Output Dryer Information.Washer Water \nTemperature ( 60 ± 5°F ):"=w343:string)
            n130 = call "DPT Worksheet DOE Audit.vi"() -> ("DOE Data Out"=w360:T13)  [unwired: 13 in, 2 out]
            n131 = Bundle By Name(cluster=w360, "Technician"=w350, "Date"=w349, "Model"=w348, "Serial"=w347, "Load Cycles"=w346, "Exhaust"=w345, "Supply Voltage"=w344, "Washer Water Temperature ( 60 ± 5°F )"=w343) -> (w362:T13)
            n132 = Bundle By Name(cluster=w356, "Heat Setting:"="Heat Setting:", "Frequency:"="Frequency:", "Dryness Setting:"="Dryness Setting:", "Washer Water \nTemperature ( 60 ± 5°F ):"="Washer Water \nTemperature ( 60 ± 5°F ):") -> (w341:T1)
            n133 = call "DPT Worksheet DOE Audit.vi"("Add?"=TRUE, "DOE Data"=w362) -> ()  [unwired: 11 in, 3 out]
            n134 = call "DPT Create Header File.vi"("Supply Voltage:"=w344, "Test_Type:"=w351, "Output Dryer Information"=w341, "Flow Computer Info Baro,BTUF,u,Z"="Flow Computer Info Baro,BTUF,u,Z") -> ("Array"=w340:string[][])  [unwired: 7 in]
            n135 = call <vilib>:"Add State(s) to Queue__jki_lib_state_machine.vi"("State(s) in (\"\")"=w365) -> ("States Out"=w364:string)  [unwired: 14 in]
            n136 = call "Calibration.vi"("Show Front Panel"=FALSE, "error in (no error)"=w359) -> ("error out"=w358:errorcluster, "Calibration Data"=w337:string[][])  [unwired: 8 in]
            n137 = Bundle By Name(cluster=w342, "Output Dryer Information.File Initialization Array"=w340, "Output Dryer Information.Calibration Array"=w337) -> (w339:T7)
            n138 = Unbundle By Name(w339) -> ("Output Dryer Information"=→"FileInit Cluster":T1)
          }
          frame "Write Globals" {
            n139 = global read "DPT Global Test Variables.vi" "Globals for Dryer Performance Test"() -> (w381:T9)
            n140 = Unbundle By Name(w378) -> ("Output Dryer Information.Model:"=w377:string, "Output Dryer Information.Ambient Temp SetPoint:"=w376:string, "Output Dryer Information.Engineer:"=w375:string, "Output Dryer Information.Technician:"=w374:string, "Output Dryer Information.Comments:"=w373:string, "Output Dryer Information.Lab ID"=w372:string, "Output Dryer Information.TR Number"=w371:string, "Output Dryer Information.Load Run Number"=w370:string, "Output Dryer Information.Test Station:"=w369:string, "Output Dryer Information.Ambient RH:"=w368:string, "Output Dryer Information.Test_Title Per TR:"=w367:string, "Output Dryer Information.Serial Number:"=w366:string)
            n141 = Unbundle By Name(w381) -> ("Test Information"=w382:T10)
            n142 = Bundle By Name(cluster=w382, "Model:"=w377, "Temperature:"=w376, "Engineer:"=w375, "Technician:"=w374, "Comments:"=w373, "Lab ID:"=w372, "TR Number:"=w371, "Test Number:"=w370, "Test Station:"=w369, "Humidity"=w368, "Test Title per TR:"=w367, "Serial Number:"=w366) -> (w380:T10)
            n143 = Bundle By Name(cluster=w381, "Test Information"=w380) -> (w379:T9)
            n144 = global write "DPT Global Test Variables.vi" "Globals for Dryer Performance Test"(w379) -> ()
            n145 = call <vilib>:"Add State(s) to Queue__jki_lib_state_machine.vi"("State(s) in (\"\")"=w385) -> ("States Out"=w384:string)  [unwired: 14 in]
          }
        }
      }
    }
    frame Error {
    }
  }
  n146 = Unbundle By Name(w4) -> ("Error Flag"=w3:bool)
  n147 = case shown="False" w3 {
    tunnel: [w387 w388] -> w2
    tunnel: w1 -> [w387 _]
    frame False {
    }
    frame True {
      n148 = local read "Unhandled Error"() -> (w388:errorcluster)
    }
  }
  "error out" <- w2
